vi "load config.vi"(8 "error in (no error)":errorcluster, 10 "TABLE":string="power_environment_monitoring", 11 "VI引用句柄":refnum<vi>) -> (0 "error out":errorcluster)   [LabVIEW 2016]
uses:
  <userlib>/_LVST/sqlite_api/Core/Select/SQLite_Select Str.vi
  <vilib>/Utility/sysdir.llb/System Directory Type.ctl
panel:
  out "数组":T1(array[cluster])
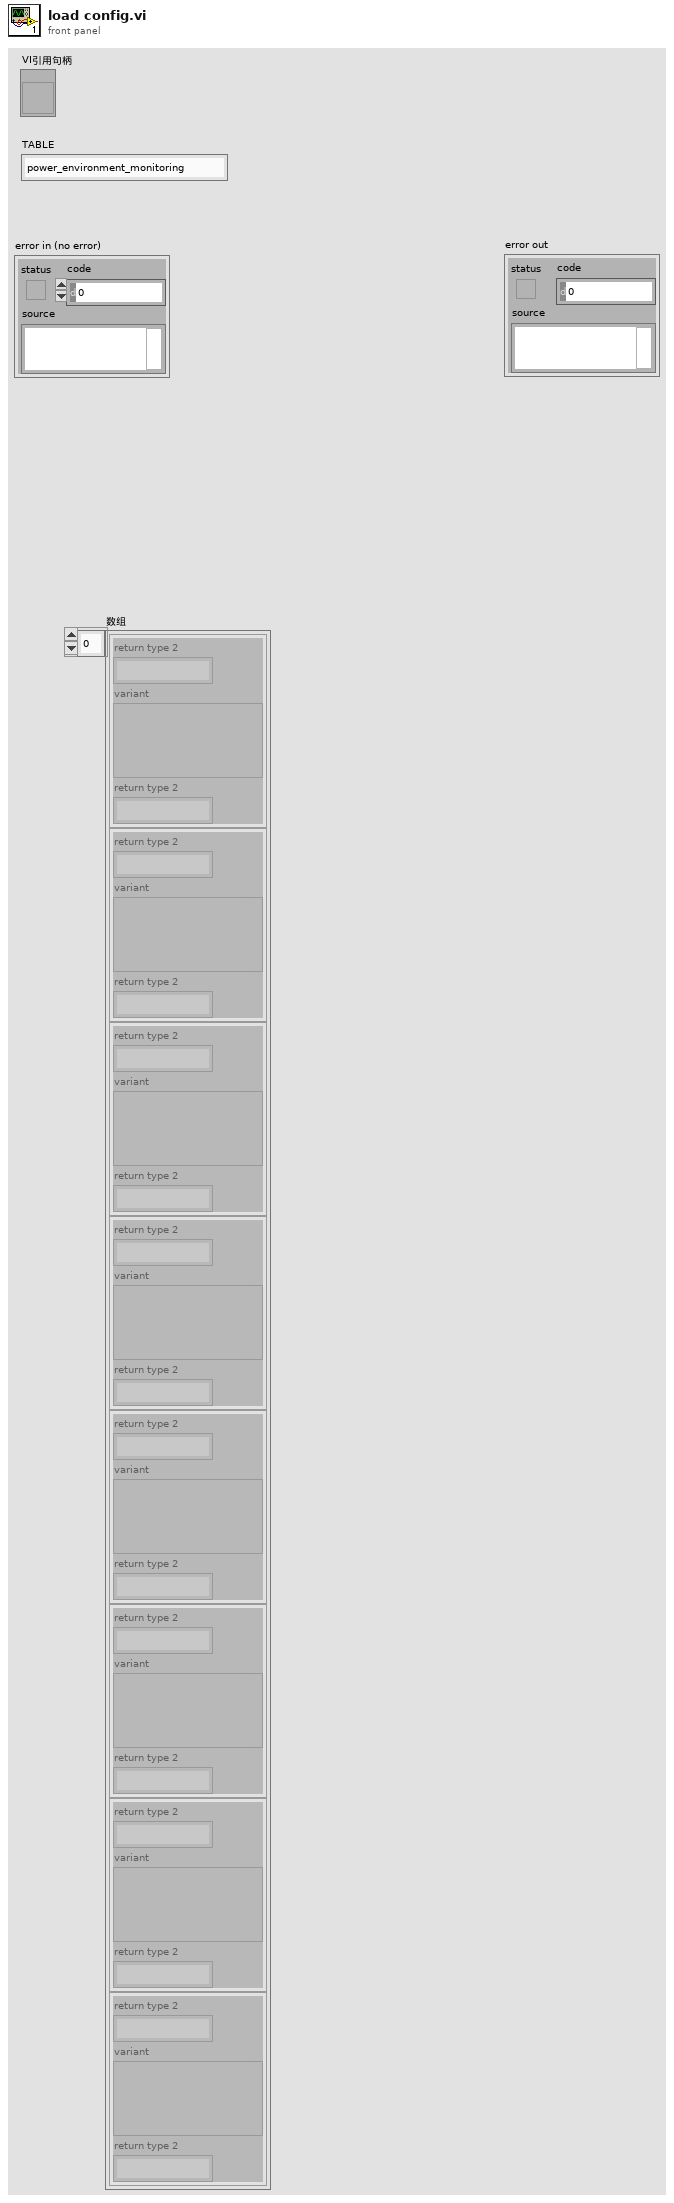
[diagram p1: front panel]
types:
  T1 = cluster{"return type 2":string, "variant":variant, "return type 2":string}[]
  T2 = typedef "System Directory Type.ctl" = i32
  T3 = cluster{"return type 2":string, variant, "return type 2":string}
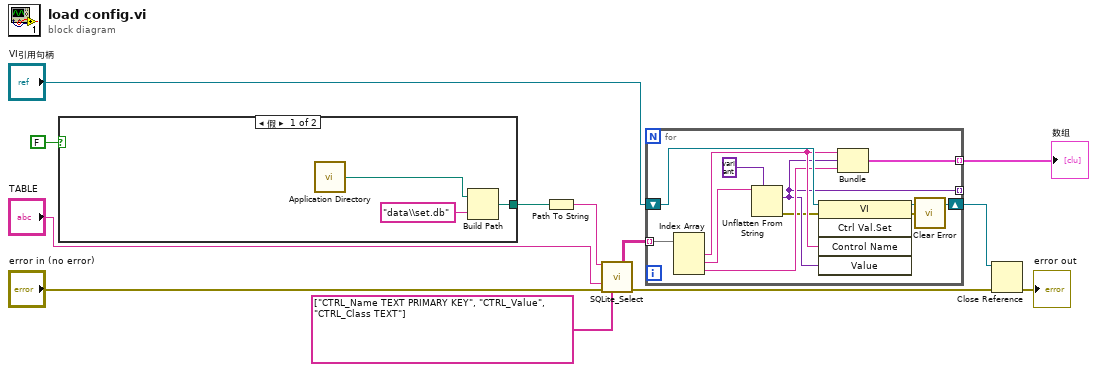
[diagram p0: block diagram]
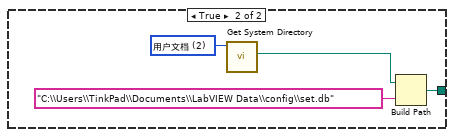
[diagram p2: hidden frame]
diagram:
  n1 = case shown="假" FALSE {
    tunnel: [w13 w16] -> w1
    frame False {
      n2 = call <vilib>:"Application Directory.vi"() -> ("Application Directory"=w15:path)
      n3 = Build Path(base path=w15, name or relative path="data\\set.db" ("名称或相对路径")) -> (appended path=w13:path)
    }
    frame True {
      w19 = T2 2 items=["用户目录"=0, "用户桌面"=1, "用户文档"=2, "用户应用程序数据"=3, "用户设置"=4, "用户临时目录"=5, "公共文档"=6, "公共应用程序数据"=7, "公共设置"=8, "公共缓存"=13, "系统核心库"=9, "系统安装库"=10, "应用程序文件"=11, "启动盘根目录"=12] ("system directory type")
      n4 = call <vilib>:"Get System Directory.vi"("system directory type"=w19) -> ("system directory"=w17:path)  [unwired: 10 in]
      n5 = Build Path(base path=w17, name or relative path="C:\\Users\\TinkPad\\Documents\\LabVIEW Data\\config\\set.db" ("名称或相对路径")) -> (appended path=w16:path)
    }
  }
  n6 = Path To String(path=w1) -> (string=w12:string)
  n7 = call-poly <userlib>:"SQLite_Select.vi"("DB Path"=w12, "Table Name"="TABLE", "error in (no error)"="error in (no error)", "Columns"=string[] ["CTRL_Name TEXT PRIMARY KEY", "CTRL_Value", "CTRL_Class TEXT"] ("Column")) -> ("Results"=w6:string[][], "error out"=w9:errorcluster)  [unwired: 8 in, 2 out]
  n8 = for {
    tunnel: w6 -> [w30] mode=indexing
    shift-right: [w27] -> w10
    shift-left: "VI引用句柄" -> [w29]
    tunnel: [w21] -> _ mode=indexing
    tunnel: [w24] -> w7 mode=indexing
    n9 = Index Array(array=w30) -> (element #1=w26:string, element #2=w23:string, element #3=w25:string)  [unwired: 3 in]
    n10 = Unflatten From String(type=variant, binary string=w23) -> (value=w21:variant, error out=w20:errorcluster)  [unwired: 3 in, 1 out]
    n11 = invoke class="VI" method="Ctrl Val.Set"(reference=w29, error in=w20, "Control Name"=w26, "Value"=w21) -> (reference out=w27:refnum<vi>, error out=w28:errorcluster)  [unwired: 1 in, 3 out]
    n12 = Bundle("return type 2"=w26, w21, "return type 2"=w25) -> (w24:T3)  [unwired: 1 in]
    n13 = call <userlib>:"Clear Error.vi"("error in (no error)"=w28) -> ()  [unwired: 4 in, 1 out]
  }
  "数组" <- w7
  n14 = Close Reference(reference=w10, error in (no error)=w9) -> (error out=→"error out":errorcluster)
